vi "Init I2C.vi"(4 "SDA GPIO":i32=4, 6 "SCL GPIO":i32=5, 7 "Bus":u8, 8 "error in (no error)":errorcluster, 10 "Baud":u32=400000 format="%.0p", 11 "VISA resource name in":refnum<visa-resource-name>) -> (0 "error out":errorcluster, 3 "VISA resource name":refnum<visa-resource-name>)   [LabVIEW 2024, in "CTIPicoVISA.lvlib"]
uses:
  CTIPicoVISA.lvlib
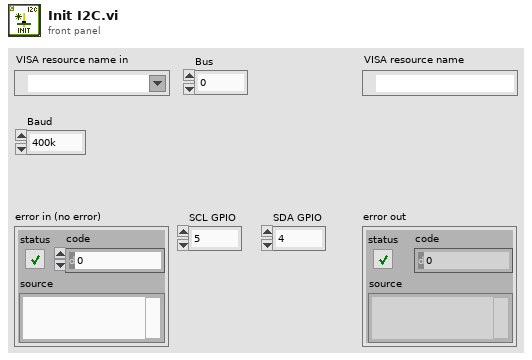
[diagram p1: front panel]
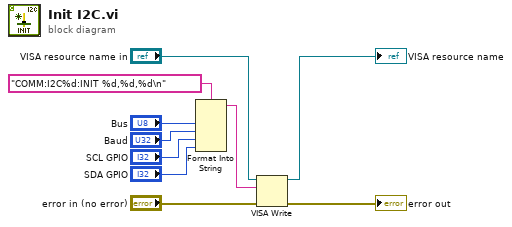
[diagram p0: block diagram]
diagram:
  n1 = Format Into String(format string="COMM:I2C%d:INIT %d,%d,%d\n", "Bus", "Baud", "SCL GPIO", "SDA GPIO") -> (resulting string=w3:string)  [unwired: 2 in, 1 out]
  n2 = VISA Write(VISA resource name="VISA resource name in", write buffer=w3, error in (no error)="error in (no error)") -> (VISA resource name out=→"VISA resource name":refnum<visa-resource-name>, error out=→"error out":errorcluster)  [unwired: 1 out]
